vi "Data.vi"(8 "error in (no error)":errorcluster, 11 "PB Msg Template in":refnum<class "Msg.lvclass">) -> (0 "error out":errorcluster, 2 "Data":T1, 3 "PB Msg Template out":refnum<class "Msg.lvclass">)   [LabVIEW 2020, in "SyncTicks.lvlib" / "Msg.lvclass"]
uses:
  Msg.lvclass
  Data.ctl
  SyncTicks.lvlib
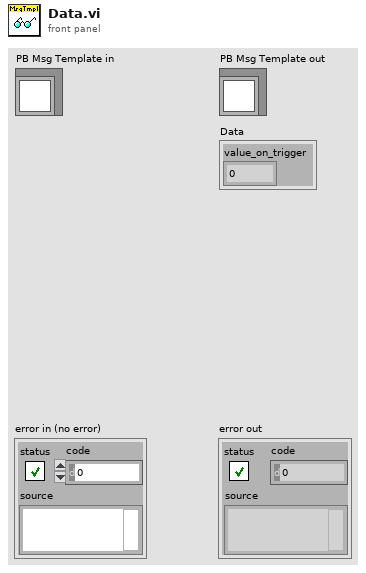
[diagram p1: front panel]
types:
  T1 = typedef "SyncTicks.lvlib/Data.ctl" = cluster{"value_on_trigger":u32}
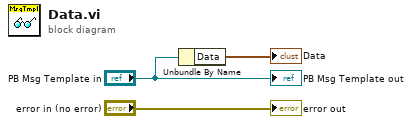
[diagram p0: block diagram]
diagram:
  n1 = Unbundle By Name("PB Msg Template in") -> ("Data"=→"Data":T1)
  "error out" <- "error in (no error)"
  "PB Msg Template out" <- "PB Msg Template in"
